vi "Shuffle.vi"(10 "Array in":T1(array[cluster]), 11 "Input":string) -> (3 "Array out":string[](array[string]))   [LabVIEW 2020]
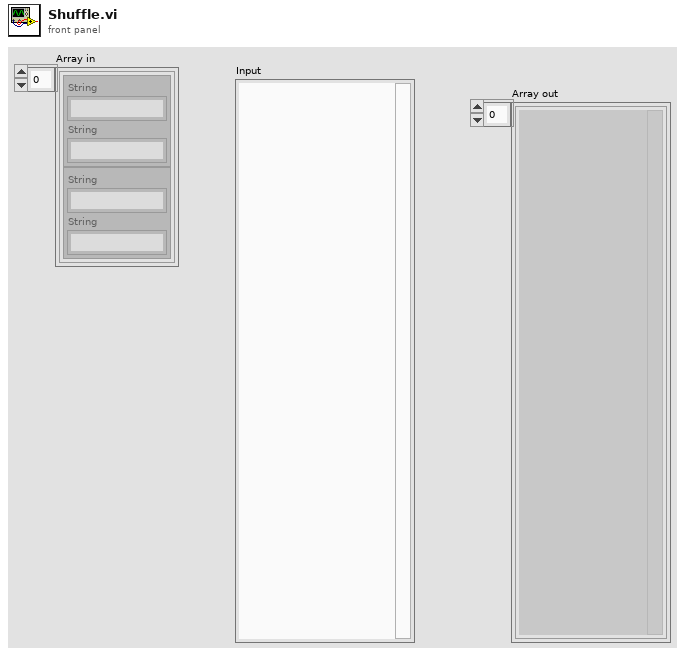
[diagram p1: front panel]
types:
  T1 = cluster{cluster{"String":string, "String":string}, cluster{"String":string, "String":string}}[]
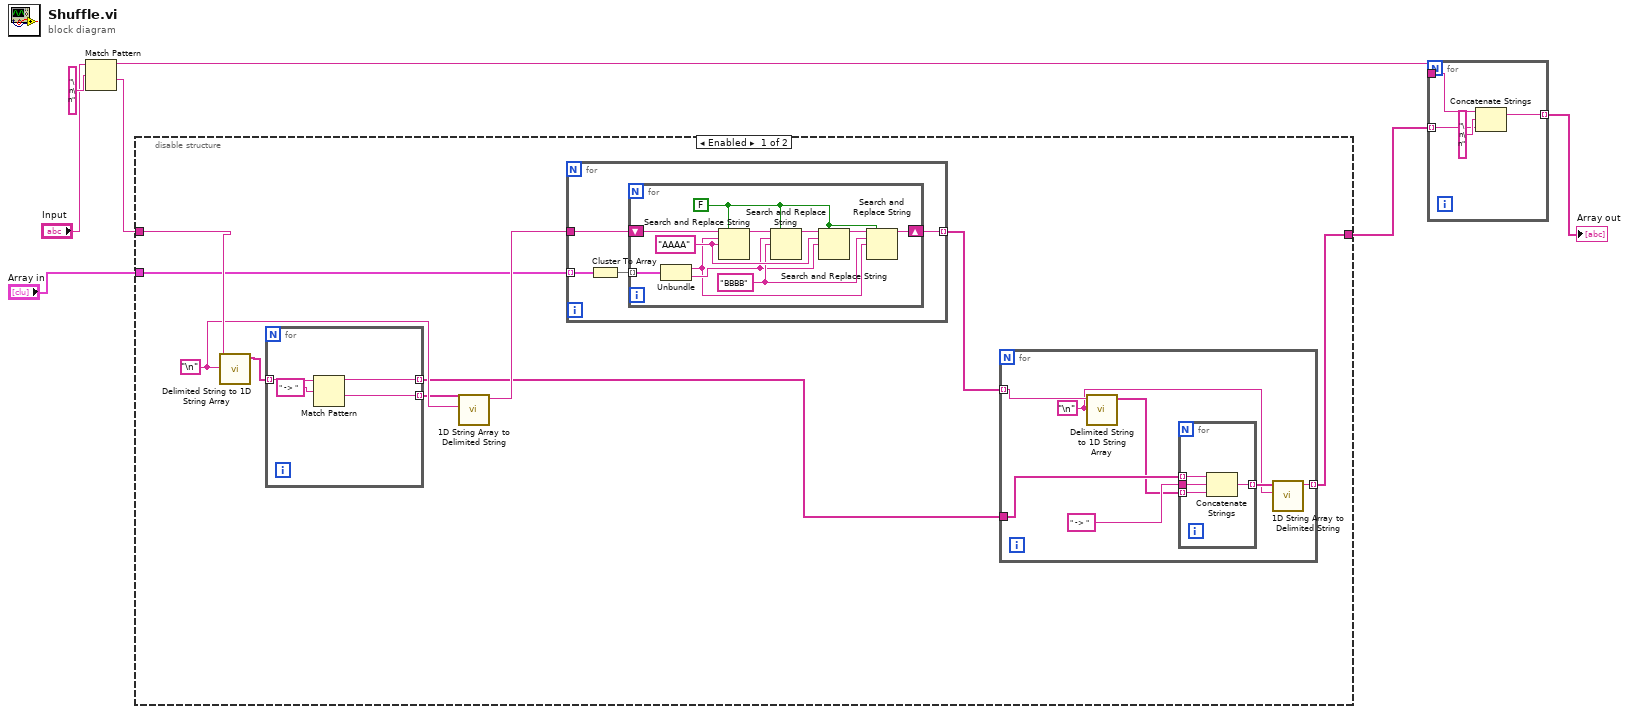
[diagram p0: block diagram]
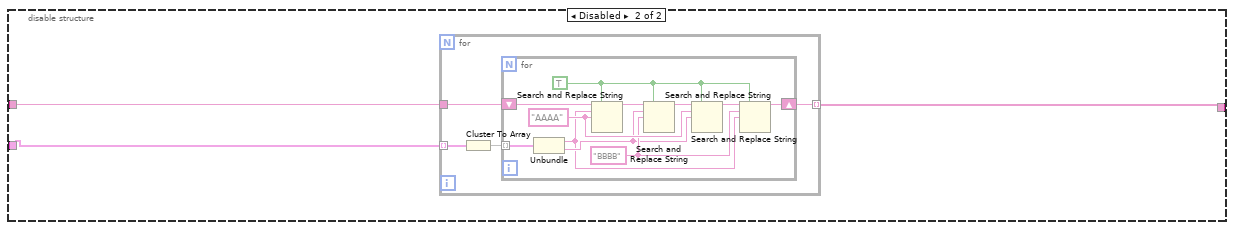
[diagram p2: hidden frame]
diagram:
  n1 = Match Pattern(string="Input", regular expression="\n\n") -> (before substring=w3:string, after substring=w4:string)  [unwired: 1 in, 2 out]
  n2 = disable-structure shown="Enabled" {
    disable-tunnel: w4 -> [w16 w48]
    disable-tunnel: [w10 w49] -> w2
    disable-tunnel: "Array in" -> [w9 w47]
    frame Enabled {
      w14 = "\n"
      n3 = call <vilib>:"Delimited String to 1D String Array.vi"("delimiter"=w14, "delimited string"=w16) -> ("string array"=w15:string[])  [unwired: 9 in]
      n4 = for {
        tunnel: w15 -> [w31] mode=indexing
        tunnel: [w29] -> w12 mode=indexing
        tunnel: [w28] -> w8 mode=indexing
        n5 = Match Pattern(string=w31, regular expression=" -> " ("delimiter")) -> (before substring=w29:string, after substring=w28:string)  [unwired: 1 in, 2 out]
      }
      n6 = call <vilib>:"1D String Array to Delimited String.vi"("delimiter"=w14, "string array"=w8) -> ("delimited string"=w13:string)  [unwired: 9 in]
      n7 = for {
        tunnel: w9 -> [w35] mode=indexing
        tunnel: w13 -> [w34]
        tunnel: [w33] -> w11 mode=indexing
        n8 = Cluster To Array(cluster=w35) -> (array=w32:cluster{"String":string, "String":string}[])
        n9 = for {
          tunnel: w32 -> [w44] mode=indexing
          shift-right: [w45] -> w33
          shift-left: w34 -> [w46]
          w36 = FALSE ("replace all? (F)")
          w42 = "BBBB" ("String")
          w43 = "AAAA"
          n10 = Unbundle(w44) -> ("String"=w40:string, "String"=w41:string)
          n11 = Search and Replace String(replace all?=w36, input string=w46, search string=w40, replace string=w43) -> (result string=w39:string)  [unwired: 4 in, 3 out]
          n12 = Search and Replace String(replace all?=w36, input string=w39, search string=w41, replace string=w42) -> (result string=w38:string)  [unwired: 4 in, 3 out]
          n13 = Search and Replace String(replace all?=w36, input string=w38, search string=w43, replace string=w41) -> (result string=w37:string)  [unwired: 4 in, 3 out]
          n14 = Search and Replace String(replace all?=w36, input string=w37, search string=w42, replace string=w40) -> (result string=w45:string)  [unwired: 4 in, 3 out]
        }
      }
      n15 = for {
        tunnel: w11 -> [w23] mode=indexing
        tunnel: w12 -> [w22]
        tunnel: [w17] -> w10 mode=indexing
        w18 = "\n"
        n16 = call <vilib>:"Delimited String to 1D String Array.vi"("delimiter"=w18, "delimited string"=w23) -> ("string array"=w20:string[])  [unwired: 9 in]
        n17 = for {
          tunnel: w22 -> [w27] mode=indexing
          tunnel: " -> " ("delimiter") -> [w26]
          tunnel: w20 -> [w25] mode=indexing
          tunnel: [w24] -> w19 mode=indexing
          n18 = Concatenate Strings(w27, w26, w25) -> (w24:string)
        }
        n19 = call <vilib>:"1D String Array to Delimited String.vi"("delimiter"=w18, "string array"=w19) -> ("delimited string"=w17:string)  [unwired: 9 in]
      }
    }
    frame Disabled {
      n20 = for {
        tunnel: w47 -> [w53] mode=indexing
        tunnel: w48 -> [w52]
        tunnel: [w51] -> w49 mode=indexing
        n21 = Cluster To Array(cluster=w53) -> (array=w50:cluster{"String":string, "String":string}[])
        n22 = for {
          tunnel: w50 -> [w61] mode=indexing
          shift-right: [w63] -> w51
          shift-left: w52 -> [w64]
          w59 = "BBBB" ("String")
          w60 = "AAAA"
          w62 = TRUE ("replace all? (F)")
          n23 = Unbundle(w61) -> ("String"=w57:string, "String"=w58:string)
          n24 = Search and Replace String(replace all?=w62, input string=w64, search string=w57, replace string=w60) -> (result string=w56:string)  [unwired: 4 in, 3 out]
          n25 = Search and Replace String(replace all?=w62, input string=w56, search string=w58, replace string=w59) -> (result string=w55:string)  [unwired: 4 in, 3 out]
          n26 = Search and Replace String(replace all?=w62, input string=w55, search string=w60, replace string=w58) -> (result string=w54:string)  [unwired: 4 in, 3 out]
          n27 = Search and Replace String(replace all?=w62, input string=w54, search string=w59, replace string=w57) -> (result string=w63:string)  [unwired: 4 in, 3 out]
        }
      }
    }
  }
  n28 = for {
    tunnel: w3 -> [w68]
    tunnel: w2 -> [w66] mode=indexing
    tunnel: [w65] -> w1 mode=indexing
    n29 = Concatenate Strings(w68, "\n\n" ("string"), w66) -> (w65:string)
  }
  "Array out" <- w1
